vi "Total Pressure Measurement.vi"(4 "error in (no error)":errorcluster, 6 "Timeout Limit":dbl format="%.2f", 7 "VISA Resource Name":refnum<visa-resource-name>="ASRL1::INSTR") -> (0 "error out":errorcluster, 1 "Timeout":bool, 2 "Total Pressure Sensitivity Factor":string, 3 "Total Pressure (torr)":dbl format="%.3e")   [LabVIEW 2021]
uses:
  Serial Support VISA.llb/Serial Actions.ctl
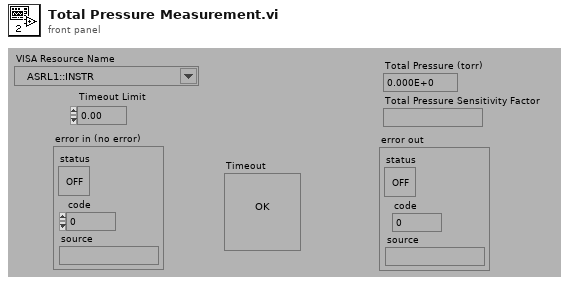
[diagram p1: front panel]
types:
  T1 = typedef "Serial Actions.ctl" = enum16{"Init", "Break", "Clear Buffer", "Write", "Read", "N Bytes", "Lock", "Unlock", "Close"}
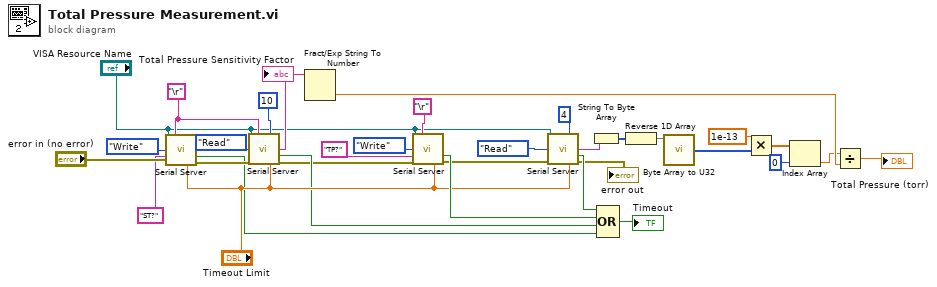
[diagram p0: block diagram]
diagram:
  w12 = "\r" ("EOT Chars (cr/lf)")
  n1 = call "Serial Server.vi"("VISA Resource Name"="VISA Resource Name", "EOT Chars (cr/lf)"=w12, "Action"=Serial_Actions."Write", "String To Send"="ST?", "error in (no error)"="error in (no error)", "Timeout Limit(sec)"="Timeout Limit") -> ("Timeout"=w13:bool, "error out"=w22:errorcluster)  [unwired: 5 in, 3 out]
  n2 = call "Serial Server.vi"("VISA Resource Name"="VISA Resource Name", "EOT Chars (cr/lf)"=w12, "Max Char to Read"=10, "Action"=Serial_Actions."Read", "error in (no error)"=w22, "Timeout Limit(sec)"="Timeout Limit") -> ("Serial Read"=w21:string, "Timeout"=w14:bool, "error out"=w9:errorcluster)  [unwired: 5 in, 2 out]
  "Total Pressure Sensitivity Factor" <- w21
  n3 = Fract/Exp String To Number(string=w21) -> (number=w16:dbl)  [unwired: 3 in, 1 out]
  n4 = call "Serial Server.vi"("VISA Resource Name"="VISA Resource Name", "EOT Chars (cr/lf)"="\r", "Action"=Serial_Actions."Write", "String To Send"="TP?", "error in (no error)"=w9, "Timeout Limit(sec)"="Timeout Limit") -> ("Timeout"=w33:bool, "error out"=w31:errorcluster)  [unwired: 5 in, 3 out]
  n5 = call "Serial Server.vi"("VISA Resource Name"="VISA Resource Name", "Max Char to Read"=4, "Action"=Serial_Actions."Read", "error in (no error)"=w31, "Timeout Limit(sec)"="Timeout Limit") -> ("Serial Read"=w26:string, "Timeout"=w32:bool, "error out"=→"error out":errorcluster)  [unwired: 6 in, 2 out]
  n6 = String To Byte Array(string=w26) -> (unsigned byte array=w25:u8[])
  n7 = Compound Arithmetic op=OR(w32, w33, w14, w13) -> (→"Timeout":bool)
  n8 = Reverse 1D Array(array=w25) -> (reversed array=w8:u8[])
  n9 = call "Byte Array to U32.vi"("Input Bytes"=w8) -> ("Output Integers"=w24:i32[])
  n10 = Multiply(x=1e-13, y=w24) -> (x*y=w4:dbl[])
  n11 = Index Array(array=w4, index=0 ("Index")) -> (element=w3:dbl)
  n12 = Divide(x=w3, y=w16) -> (x/y=→"Total Pressure (torr)":dbl)
